vi "Empty Front Panel And Diagram(冲突时的文件备份2013-05-03 09-31-55).vi"   [LabVIEW 2012]
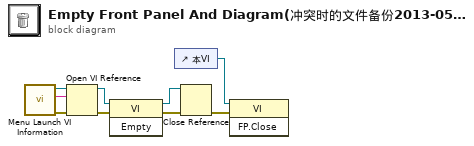
[diagram p0: block diagram]
diagram:
  n1 = call <vilib>:"Menu Launch VI Information.vi"() -> ("error out"=w7:errorcluster, "Menu Launch:VI"=w5:string, "Menu Launch:App"=w6:refnum<vi>)  [unwired: 9 in]
  n2 = Open VI Reference(application reference (local)=w6, vi path=w5, error in (no error)=w7) -> (vi reference=w4:refnum<vi>, error out=w2:errorcluster)  [unwired: 3 in]
  n3 = invoke class="VI" method="Empty"(reference=w4, error in=w2) -> (reference out=w3:refnum<vi>, error out=w1:errorcluster)  [unwired: 1 in, 1 out]
  n4 = control-ref of="本VI"() -> (w9:refnum<vi>)
  n5 = Close Reference(reference=w3, error in (no error)=w1) -> (error out=w8:errorcluster)
  n6 = invoke class="VI" method="FP.Close"(reference=w9, error in=w8) -> ()  [unwired: 1 in, 3 out]
